vi "hokuyo_closestObject.vi"(1 "Current stepper angle":dbl, 2 "Array":cluster{"Magnitude":dbl, "Direction":dbl}[](array[cluster])) -> (0 "Target Direction":dbl)   [LabVIEW 2014]
panel:
  out "Object Distance":dbl
  in  "stop":bool
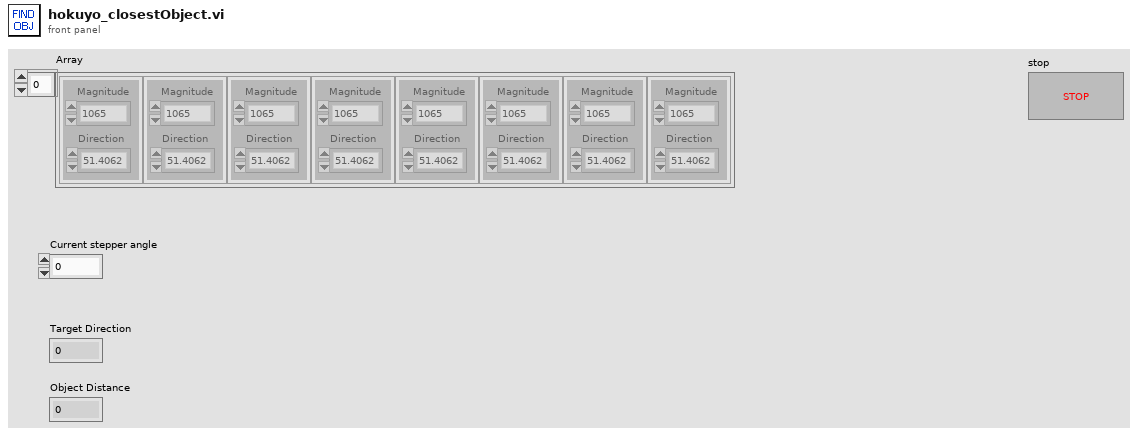
[diagram p1: front panel]
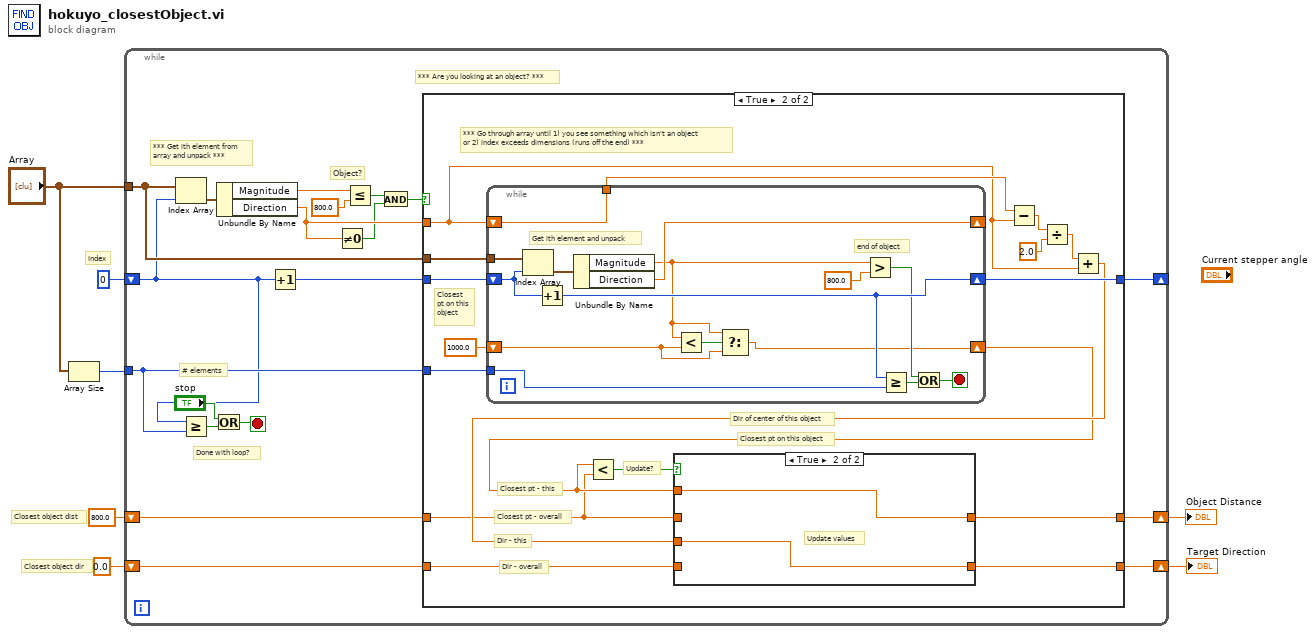
[diagram p0: block diagram]
diagram:
  # "Index"
  # "Closest object dir"
  # "Closest object dist"
  n1 = Array Size(array="Array") -> (size(s)=w2:i32)
  n2 = while {
    tunnel: "Array" -> [w25]
    shift-right: [w26] -> _
    shift-left: 0 -> [w13]
    shift-right: [w16] -> w4
    shift-left: 800.0 -> [w23]
    shift-right: [w15] -> w3
    shift-left: 0.0 ("Largest Hole Direction") -> [w24]
    tunnel: w2 -> [w18]
    stop <- w22 stop-if-true
    # "# elements"
    # "Object?"
    # "Done with loop?"
    # "*** Are you looking at an object? ***"
    # "*** Get ith element from \narray and unpack ***"
    n3 = Index Array(array=w25, index=w13) -> (element=w12:cluster{"Magnitude":dbl, "Direction":dbl})
    n4 = Greater Or Equal?(x=w13, y=w18) -> (x >= y?=w21:bool)
    n5 = Or(x="stop", y=w21) -> (x .or. y?=w22:bool)
    n6 = Unbundle By Name(w12) -> ("Magnitude"=w17:dbl, "Direction"=w11:dbl)
    n7 = Increment(x=w13) -> (x+1=w14:i32)
    n8 = Not Equal To 0?(x=w11) -> (x != 0?=w10:bool)
    n9 = Less Or Equal?(x=w17, y=800.0) -> (x <= y?=w9:bool)
    n10 = And(x=w9, y=w10) -> (x .and. y?=w8:bool)
    n11 = case shown="True" w8 {
      tunnel: w14 -> [w29 w46]
      tunnel: [w29 w40] -> w26
      tunnel: w25 -> [_ w45]
      tunnel: w11 -> [_ w30]
      tunnel: w24 -> [w28 w36]
      tunnel: w23 -> [w27 w32]
      tunnel: [w28 w42] -> w15
      tunnel: [w27 w34] -> w16
      tunnel: w18 -> [_ w39]
      frame False {
        # "*** Keep looking for the beginning of a hole ***"
      }
      frame True {
        # "Update?"
        # "Dir - overall"
        # "Dir - this"
        # "Closest pt - overall"
        # "Closest pt - this"
        # "Closest pt on this object"
        # "Closest\npt on this\nobject"
        # "Dir of center of this object"
        # "*** Go through array until 1) you see something which isn't an object \nor 2) index exceeds dimensions (runs off the end) ***"
        n12 = while {
          tunnel: w45 -> [w65]
          shift-right: [w60] -> w40
          shift-left: w46 -> [w62]
          tunnel: w39 -> [w59]
          shift-right: [w57] -> _
          shift-left: w30 -> [w56]
          tunnel: [w56] -> w38
          shift-right: [w51] -> w33
          shift-left: 1000.0 -> [w53]
          stop <- w61 stop-if-true
          # "end of object"
          # "Get ith element and unpack"
          n13 = Index Array(array=w65, index=w62) -> (element=w63:cluster{"Magnitude":dbl, "Direction":dbl})
          n14 = Increment(x=w62) -> (x+1=w60:i32)
          n15 = Unbundle By Name(w63) -> ("Magnitude"=w52:dbl, "Direction"=w57:dbl)
          n16 = Less?(x=w52, y=w53) -> (x < y?=w54:bool)
          n17 = Select(t=w52, s=w54, f=w53) -> (s? t:f=w51:dbl)
          n18 = Greater?(x=w52, y=800.0) -> (0:w55:bool)
          n19 = Greater Or Equal?(x=w60, y=w59) -> (x >= y?=w58:bool)
          n20 = Or(x=w55, y=w58) -> (x .or. y?=w61:bool)
        }
        n21 = Less?(x=w33, y=w32) -> (x < y?=w31:bool)
        n22 = Subtract(x=w38, y=w30) -> (x-y=w41:dbl)
        n23 = Divide(x=w41, y=2.0) -> (x/y=w43:dbl)
        n24 = Add(x=w43, y=w30) -> (x+y=w37:dbl)
        n25 = case shown="True" w31 {
          tunnel: w37 -> [_ w50]
          tunnel: w36 -> [w48 _]
          tunnel: [w48 w50] -> w42
          tunnel: w33 -> [_ w49]
          tunnel: w32 -> [w47 _]
          tunnel: [w47 w49] -> w34
          frame False {
            # "Keep old values"
          }
          frame True {
            # "Update values"
          }
        }
      }
    }
  }
  "Object Distance" <- w4
  "Target Direction" <- w3
